vi "FullCommunicator.vi"() -> ()   [LabVIEW 2014]
uses:
  <vilib>/Instr/_visa.llb/VISA Set IO Buffer Mask.ctl
  <vilib>/Instr/_visa.llb/VISA Configure Serial Port (Instr).vi
panel:
  out "Distance":sgl
  out "PWM":sgl(graph)
  out "Omega Esum":sgl
  in  "adr":u8[](array[numeric])
  out "ANgleOutSignal":sgl
  out "OmegaOutSignal":sgl
  out "concatenated string":string
  in  "Value":sgl
  out "PidAngleDst":dbl
  out "PidOmegaKd":dbl
  out "PidOmegaKi":dbl
  out "PidOmegaKp":dbl
  out "PidAngleKd":dbl
  out "PidAngleKi":dbl
  out "PidAngleKp":dbl
  out "Omega Right":sgl(graph)
  out "Omega Left":sgl(graph)
  out "tim":dbl
  in  "Wyœlij":bool
  out "Kalman Q_Angle":dbl
  out "Raw Angle":sgl(graph)
  out "Filtered Angle":sgl(graph)
  out "Kalman R_Measure":dbl
  out "return count":u32
  in  "VISA resource name":refnum<visa-resource-name>
  in  "stop rec":bool
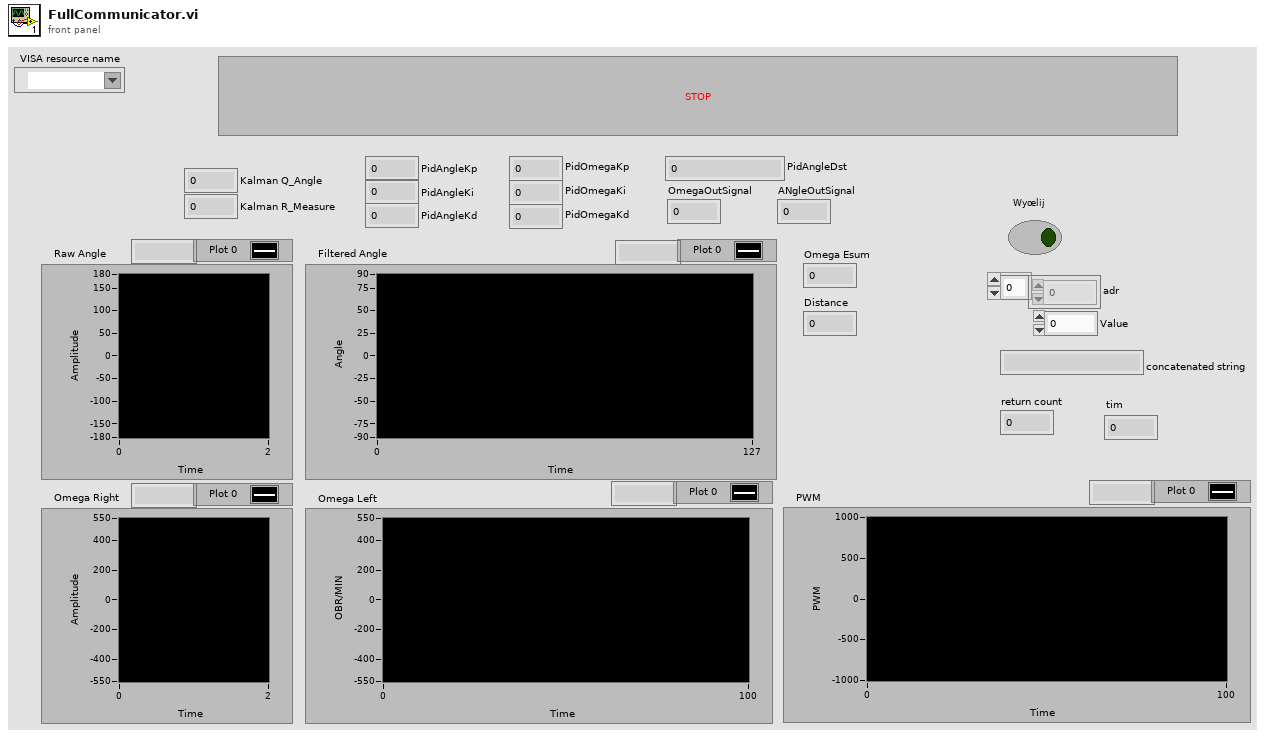
[diagram p1: front panel]
types:
  T1 = typedef "VISA Set IO Buffer Mask.ctl" = u16
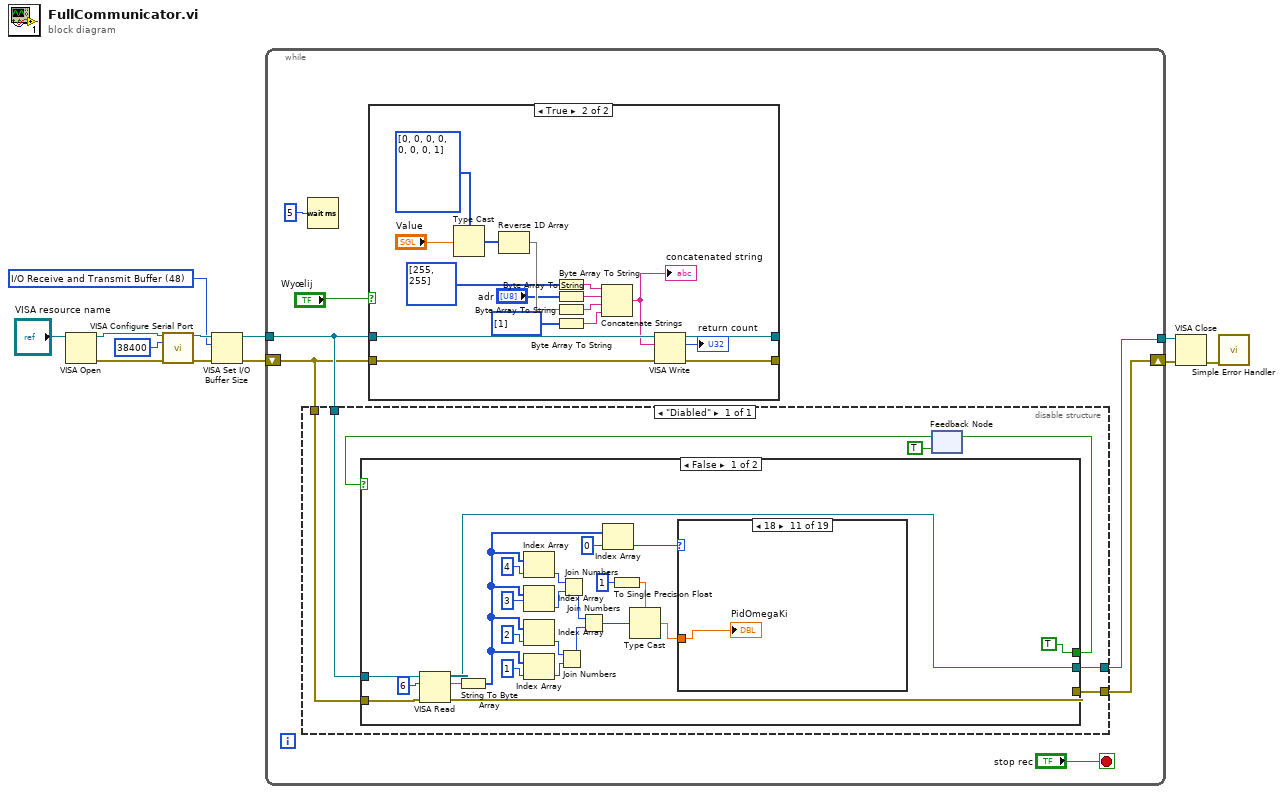
[diagram p0: block diagram]
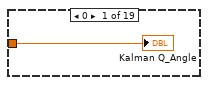
[diagram p2: hidden frame]
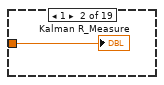
[diagram p3: hidden frame]
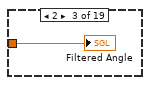
[diagram p4: hidden frame]
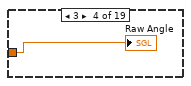
[diagram p5: hidden frame]
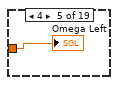
[diagram p6: hidden frame]
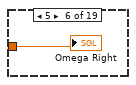
[diagram p7: hidden frame]
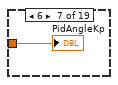
[diagram p8: hidden frame]
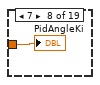
[diagram p9: hidden frame]
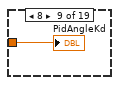
[diagram p10: hidden frame]
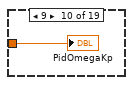
[diagram p11: hidden frame]
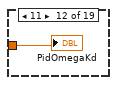
[diagram p12: hidden frame]
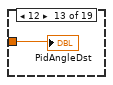
[diagram p13: hidden frame]
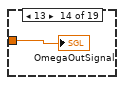
[diagram p14: hidden frame]
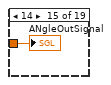
[diagram p15: hidden frame]
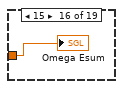
[diagram p16: hidden frame]
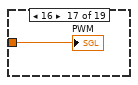
[diagram p17: hidden frame]
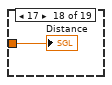
[diagram p18: hidden frame]
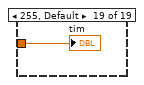
[diagram p19: hidden frame]
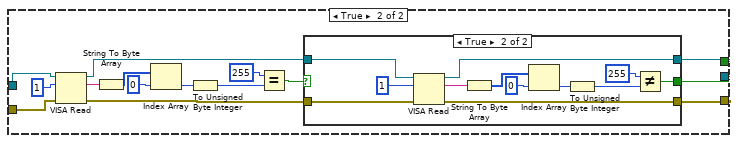
[diagram p20: hidden frame]
diagram:
  w8 = T1 48 items=["I/O Receive Buffer"=16, "I/O Transmit Buffer"=32, "I/O Receive and Transmit Buffer"=48] ("Mask")
  n1 = VISA Open(VISA resource name="VISA resource name") -> (VISA resource name=w12:refnum<visa-resource-name>, error out=w9:errorcluster)  [unwired: 4 in]
  n2 = call-poly "VISA Configure Serial Port"("VISA resource name"=w12, "baud rate (9600)"=u32 38400, "error in (no error)"=w9) -> ("VISA resource name out"=w11:refnum<visa-resource-name>, "error out"=w10:errorcluster)  [unwired: 11 in]
  n3 = VISA Set I/O Buffer Size(VISA resource name=w11, mask (16)=w8, error in (no error)=w10) -> (VISA resource name out=w4:refnum<visa-resource-name>, error out=w5:errorcluster)  [unwired: 1 in]
  n4 = while {
    tunnel: w4 -> [w17]
    tunnel: [w14] -> w2
    shift-right: [w15] -> w1
    shift-left: w5 -> [w16]
    stop <- "stop rec" stop-if-true
    n5 = disable-structure shown="\"Diabled\"" {
      disable-tunnel: w17 -> [w23]
      disable-tunnel: w16 -> [w22]
      disable-tunnel: [w21] -> w15
      disable-tunnel: [w20] -> w14
      frame condition #0 (active) {
        n6 = feedback #1(TRUE) -> (w26:bool)
        n7 = case shown="False" w26 {
          tunnel: w23 -> [w31 w84]
          tunnel: w22 -> [w30 w83]
          tunnel: [w28 w72] -> w21
          tunnel: [w29 w74] -> w20
          tunnel: [TRUE w70] -> w25
          frame False {
            n8 = VISA Read(VISA resource name=w31, byte count=u32 6, error in (no error)=w30) -> (VISA resource name out=w29:refnum<visa-resource-name>, read buffer=w49:string, error out=w28:errorcluster)  [unwired: 1 out]
            n9 = String To Byte Array(string=w49) -> (unsigned byte array=w42:u8[])
            n10 = Index Array(array=w42, index=4) -> (element=w41:u8)
            n11 = Index Array(array=w42, index=3) -> (element=w40:u8)
            n12 = Index Array(array=w42, index=2) -> (element=w39:u8)
            n13 = Index Array(array=w42, index=1) -> (element=w38:u8)
            n14 = Join Numbers(hi=w39, lo=w38) -> ((hi.lo)=w36:u16)
            n15 = Join Numbers(hi=w41, lo=w40) -> ((hi.lo)=w37:u16)
            n16 = Join Numbers(hi=w37, lo=w36) -> ((hi.lo)=w35:u32)
            n17 = Index Array(array=w42, index=0) -> (element=w47:u8)
            n18 = To Single Precision Float(number=1 ("index")) -> (single precision float=w33:sgl)
            n19 = Type Cast(type=w33, x=w35) -> (*(type *) &x=w32:sgl)
            n20 = case shown="18" w47 {
              tunnel: w32 -> [w51 w52 w53 w54 w55 w56 w57 w58 w59 w60 w61 w62 w63 w64 w65 w66 w67 w68 w69]
              frame 0 {
                "Kalman Q_Angle" <- w51
              }
              frame 1 {
                "Kalman R_Measure" <- w52
              }
              frame 2 {
                "Filtered Angle" <- w53
              }
              frame 3 {
                "Raw Angle" <- w54
              }
              frame 4 {
                "Omega Left" <- w55
              }
              frame 5 {
                "Omega Right" <- w56
              }
              frame 6 {
                "PidAngleKp" <- w57
              }
              frame 7 {
                "PidAngleKi" <- w58
              }
              frame 8 {
                "PidAngleKd" <- w59
              }
              frame 9 {
                "PidOmegaKp" <- w60
              }
              frame 18 {
                "PidOmegaKi" <- w61
              }
              frame 11 {
                "PidOmegaKd" <- w62
              }
              frame 12 {
                "PidAngleDst" <- w63
              }
              frame 13 {
                "OmegaOutSignal" <- w64
              }
              frame 14 {
                "ANgleOutSignal" <- w65
              }
              frame 15 {
                "Omega Esum" <- w66
              }
              frame 16 {
                "PWM" <- w67
              }
              frame 17 {
                "Distance" <- w68
              }
              frame 255, Default {
                "tim" <- w69
              }
            }
          }
          frame True {
            n21 = VISA Read(VISA resource name=w84, byte count=u32 1, error in (no error)=w83) -> (VISA resource name out=w75:refnum<visa-resource-name>, read buffer=w78:string, error out=w73:errorcluster)  [unwired: 1 out]
            n22 = String To Byte Array(string=w78) -> (unsigned byte array=w81:u8[])
            n23 = Index Array(array=w81, index=0) -> (element=w79:u8)
            n24 = To Unsigned Byte Integer(number=w79) -> (unsigned 8bit integer=w76:u8)
            n25 = Equal?(x=u8 255, y=w76) -> (x = y?=w71:bool)
            n26 = case shown="True" w71 {
              selector: w71 -> [w86 _]
              tunnel: w75 -> [w87 w93]
              tunnel: [w87 w92] -> w74
              tunnel: w73 -> [w88 w91]
              tunnel: [w88 w90] -> w72
              tunnel: [w85 w89] -> w70
              frame False {
                n27 = Not(x=w86) -> (.not. x?=w85:bool)
              }
              frame True {
                n28 = VISA Read(VISA resource name=w93, byte count=u32 1, error in (no error)=w91) -> (VISA resource name out=w92:refnum<visa-resource-name>, read buffer=w96:string, error out=w90:errorcluster)  [unwired: 1 out]
                n29 = String To Byte Array(string=w96) -> (unsigned byte array=w99:u8[])
                n30 = Index Array(array=w99, index=0) -> (element=w97:u8)
                n31 = To Unsigned Byte Integer(number=w97) -> (unsigned 8bit integer=w94:u8)
                n32 = Not Equal?(x=u8 255, y=w94) -> (x != y?=w89:bool)
              }
            }
          }
        }
        n33 = feedback-in #1(w25) -> ()
      }
    }
    n34 = Wait (ms)(milliseconds to wait=u32 5) -> ()  [unwired: 1 out]
    n35 = case shown="True" "Wyœlij" {
      tunnel: w16 -> [w101 w119]
      tunnel: w17 -> [w102 w118]
      tunnel: [w101 w117] -> _
      tunnel: [w102 w116] -> _
      frame False {
      }
      frame True {
        n36 = Type Cast(type=u8[] [0, 0, 0, 0, 0, 0, 0, 1] ("Command"), x="Value") -> (*(type *) &x=w114:u8[])
        n37 = Reverse 1D Array(array=w114) -> (reversed array=w106:u8[])
        n38 = Byte Array To String(unsigned byte array=u8[] [255, 255]) -> (string=w105:string)
        n39 = Byte Array To String(unsigned byte array="adr") -> (string=w110:string)
        n40 = Byte Array To String(unsigned byte array=w106) -> (string=w109:string)
        n41 = Byte Array To String(unsigned byte array=u8[] [1]) -> (string=w108:string)
        n42 = Concatenate Strings(w105, w110, w109, w108) -> (w111:string)
        "concatenated string" <- w111
        n43 = VISA Write(VISA resource name=w118, write buffer=w111, error in (no error)=w119) -> (VISA resource name out=w116:refnum<visa-resource-name>, return count=→"return count":u32, error out=w117:errorcluster)
      }
    }
  }
  n44 = VISA Close(VISA resource name=w2, error in (no error)=w1) -> (error out=w3:errorcluster)
  n45 = call <vilib>:"Simple Error Handler.vi"("error in (no error)"=w3) -> ()  [unwired: 4 in, 5 out]
